vi "Monitor.vi"() -> ()   [LabVIEW 2019]
uses:
  <instrlib>/Siemens ELAN/Message Header.ctl
  <instrlib>/Siemens ELAN/Channel Status.ctl
  <instrlib>/Siemens ELAN/Unit Dimensions.ctl
  <instrlib>/Siemens ELAN/Measured variables.ctl
  <instrlib>/Siemens ELAN/Siemens ELAN.lvlib
panel:
  out "Measured variable":T1
  in  "Source Address":u8=208 format="%.0x"
  in  "Target Address":u8=16 format="%.0x"
  in  "New Name":string
  in  "VISA resource name":refnum<visa-resource-name>="OXYMAT"
  in  "Set Clock":bool
  in  "VISA Timeout Value":u32=200
  out "Channel Name":string
  out "Measurement":cluster{"Measured value":dbl, "Dimension":T2}={"Measured value"=nan, "Dimension"=enum."Unknown (0)"} {"Measured value" format="%#_6f"}
  in  "Broadcast ON?":bool
  out "Maintenance Requests":T3(array[ring])
  in  "Reset":bool
  in  "Remote ON?":bool
  in  "Maintenance ON?":bool
  out "Faults/Errors":T4(array[ring])
  out "time stamp":timestamp format="%<%Y-%m-%dT%H:%M:%S>T"
  out "Channel":T5
  out "Channel Type":T6(ring)
  out "x-y":u32
  in  "milliseconds to wait":u32
  in  "stop":bool
  out "Success":bool
  out "Message Header":T7 {"Source Address" format="%.0x"; "Target Address" format="%.0x"}
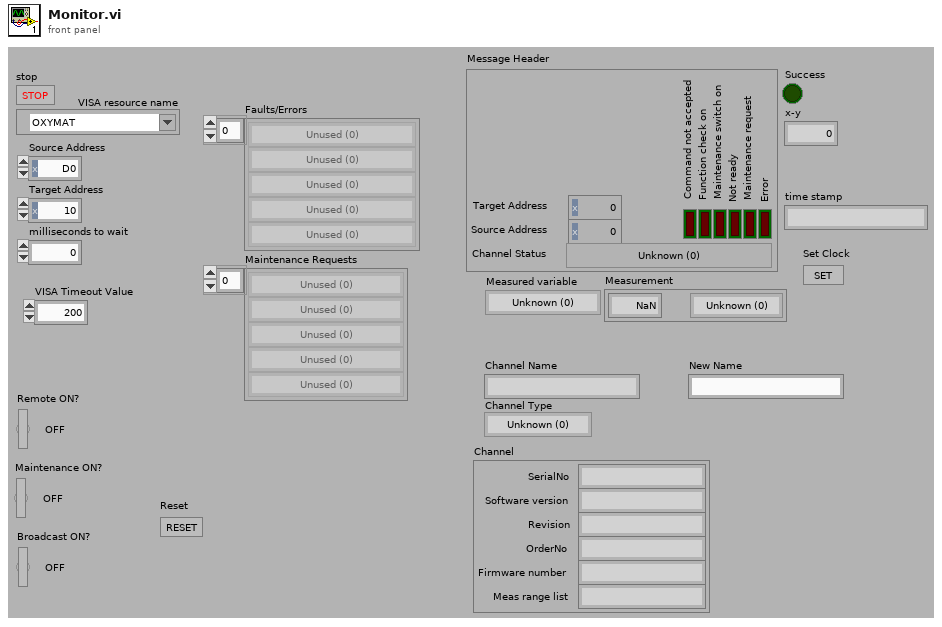
[diagram p1: front panel]
types:
  T1 = typedef "Siemens ELAN.lvlib/Measured variables.ctl" = enum8{"Unknown (0)", "No component", "CO", "CO2", "CH4", "C6H14", "SO2", "NO", "NO2", "CHClF2 (R22)", "C3H8", "C4H10", "O2", "C5H12", "HC", "Pressure", "pH", "Temperature", "C2H4", "C2H2", "C3H6", "C4H6", "C4H8", "C2H6", "NH3", "N2O", "C6H6", "SF6", "CH3OH", "C2H5OH", "CH2Cl2", "C2H4Cl2", "CH3Cl", "C2H4O", "H2O (vapor)", "G/l", "Unknown (36)", "Unknown (37)", "Unknown (38)", "Unknown (39)", "Unknown (40)", "Unknown (41)", "Unknown (42)", "Unknown (43)", "Unknown (44)", "Unknown (45)", "Unknown (46)", "Unknown (47)", "Unknown (48)", "Unknown (49)", "Unknown (50)", "Unknown (51)", "Unknown (52)", "Unknown (53)", "Unknown (54)", "Unknown (55)", "Unknown (56)", "Unknown (57)", "Unknown (58)", "Unknown (59)", "Unknown (60)", "Unknown (61)", "Unknown (62)", "Unknown (63)", "Unknown (64)", "Unknown (65)", "Unknown (66)", "Unknown (67)", "Unknown (68)", "Unknown (69)", "Unknown (70)", "Unknown (71)", "Unknown (72)", "Unknown (73)", "Unknown (74)", "Unknown (75)", "Unknown (76)", "Unknown (77)", "Unknown (78)", "Unknown (79)", "Unknown (80)", "Unknown (81)", "Unknown (82)", "Unknown (83)", "Unknown (84)", "Unknown (85)", "Unknown (86)", "Unknown (87)", "Unknown (88)", "Unknown (89)", "Unknown (90)", "Unknown (91)", "Unknown (92)", "Unknown (93)", "Unknown (94)", "Unknown (95)", "Unknown ((96)", "Unknown (97)", "Unknown (98)", "Unknown (99)", "Ambient Pressure", "Unknown (>100)"}
  T2 = typedef "Siemens ELAN.lvlib/Unit Dimensions.ctl" = enum8{"Unknown (0)", "Pure number", "ppm", "ppb", "vpm", "vpm C1", "vpm C3", "vpm C6", "mg C/m^3", "mg/m^3", "%", "% v/v", "% of range", "% saturation", "%/°C", "%/K", "% w/w", "mV/pH", "mV/mbar", "nA/mbar", "S/m", "S/cm", "mS/m", "mS/cm", "uS/m", "uS/cm", "s", "min", "hr", "pA", "mA", "uV", "mV", "V", "mbar", "hPa", "ml/min", "kohm", "MOhm", "S", "°C", "Hz", "pH", "ug/l", "mg/l", "l/min", "uA", "mg/dm^3", "kPa", "kohm*cm", "MOhm*cm", "°", "Unknown (>51)"}
  T3 = enum8{"Unused (0)", "Cal Tolerance Violated", "Signal Too High With Zero Adj", "Signal Too Low With Span", "Set Clock", "Microflow Sensor Drift", "Display Temperature", "Analyzer Temperature", "Measuring Head Temperature", "External Request"}[]
  T4 = enum8{"Unused (0)", "Param Memory", "Chopper/Magnetic Field", "Microflow Sensor", "External Fault", "AnalyzerTemperature", "Field Device Heater", "Measuring Head Temperature", "Pressure Sensor", "Signal Too Large", "Unused (S10)", "Reference Gas Supply", "Main Power", "Unused (S13)", "Measured Value > Full Scale", "Calibration Aborted", "Low Sample Flow "}[]
  T5 = cluster{"SerialNo":string, "Software version":string, "Revision":string, "OrderNo":string, "Firmware number":string, "Meas range list":string}
  T6 = enum8{"Unknown (0)", "ULTRAMAT 6", "OXYMAT 6", "FIDAMAT 6", "ULTRAMAT 23", "SIPAN 34", "Unknown (6)", "CALOMAT 6", "Unknown (>7)"}
  T7 = typedef "Siemens ELAN.lvlib/Message Header.ctl" = cluster{"Target Address":u8, "Source Address":u8, "Error":bool, "Maintenance request":bool, "Not ready":bool, "Maintenance switch on":bool, "Function check on":bool, "Command not accepted":bool, "Channel Status":T8}
  T8 = typedef "Siemens ELAN.lvlib/Channel Status.ctl" = enum8{"Unknown (0)", "Warm-up", "Pause", "Standby", "Measure", "Zero calibration", "Adjust component slope", "Unknown (7)", "Adjust curve dip", "Adjust linearization sensitivity", "Adjust temperature compensation", "Adjust pressure compensation", "Adjust linearization zero", "Adjust flow sensor", "Autocal", "Adjust phase", "Zero calibration of O2 sensor", "Synchronous zero calibration", "Purging for synchronous zero calibration", "Adjust analog output", "Adjust analog input", "Cleaning", "Unknown (>21)"}
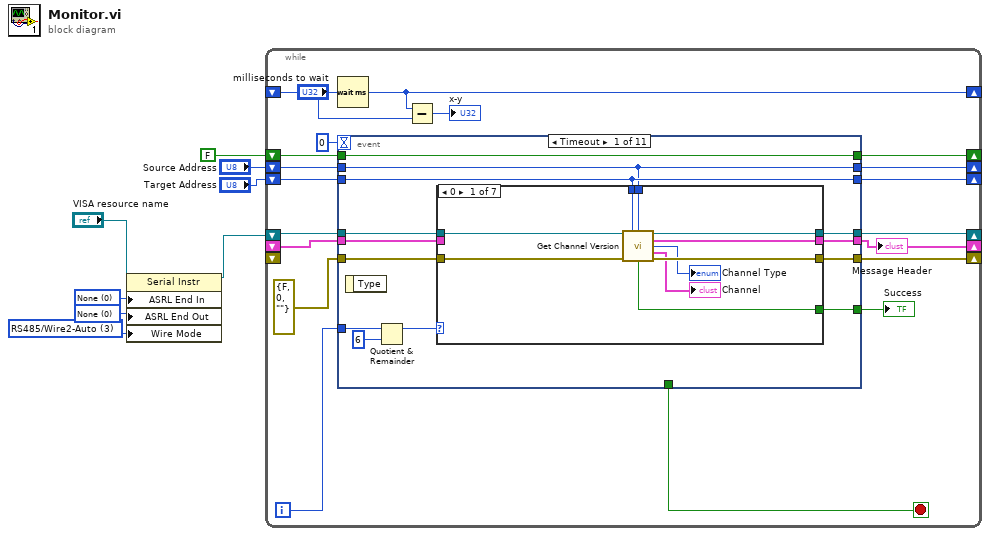
[diagram p0: block diagram]
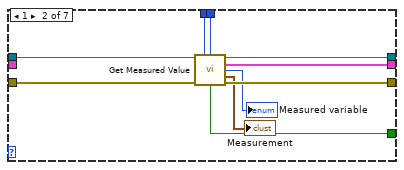
[diagram p2: hidden frame]
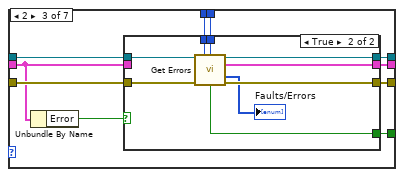
[diagram p3: hidden frame]
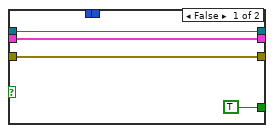
[diagram p4: hidden frame]
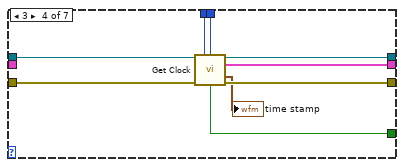
[diagram p5: hidden frame]
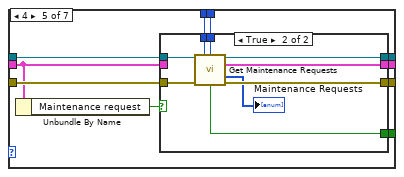
[diagram p6: hidden frame]
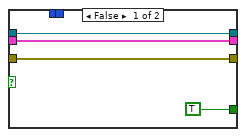
[diagram p7: hidden frame]
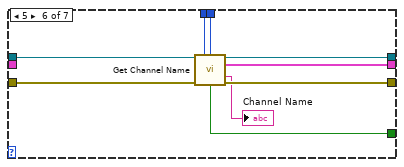
[diagram p8: hidden frame]
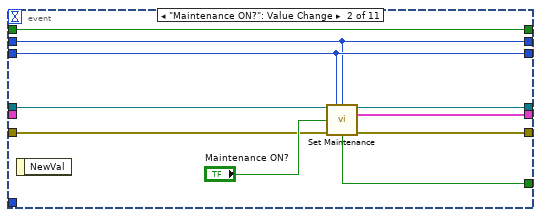
[diagram p10: hidden frame]
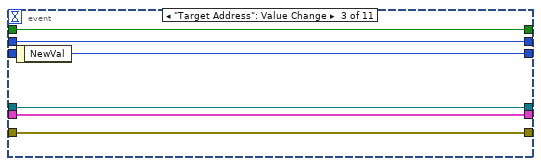
[diagram p11: hidden frame]
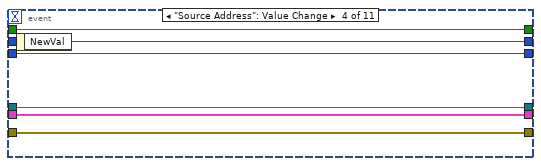
[diagram p12: hidden frame]
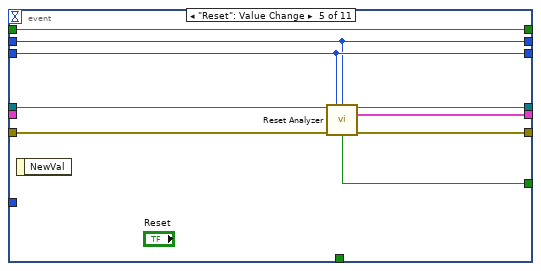
[diagram p13: hidden frame]
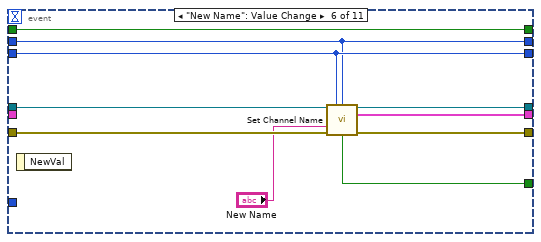
[diagram p14: hidden frame]
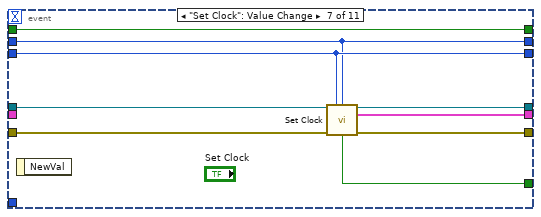
[diagram p15: hidden frame]
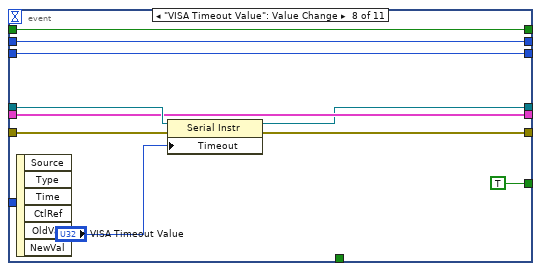
[diagram p16: hidden frame]
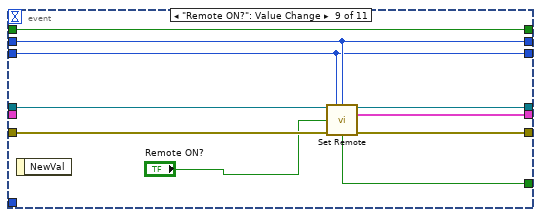
[diagram p17: hidden frame]
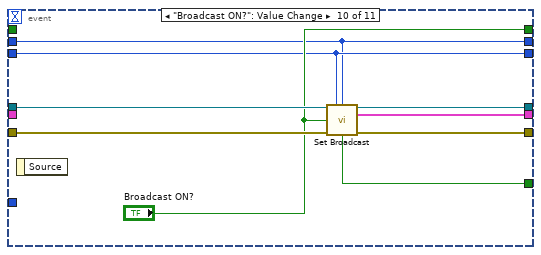
[diagram p18: hidden frame]
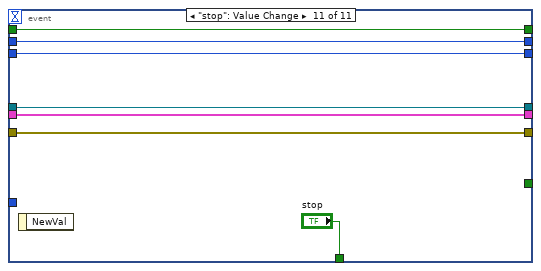
[diagram p19: hidden frame]
diagram:
  w3 = u16 0 items=["None", "Last Bit", "TermChar"] ("Serial Settings:End Mode for Reads")
  w4 = u16 0 items=["None", "Last Bit", "TermChar", "Break"] ("Serial Settings:End Mode for Writes")
  w5 = i16 3 items=["Unknown"=-1, "RS485/Wire4"=0, "RS485/Wire2-EchoDTR"=1, "RS485/Wire2-CtrlDTR"=2, "RS485/Wire2-Auto"=3, "RS232/DTE"=128, "RS232/DCE"=129, "RS232/AUTO"=130] ("Serial Settings:Wire Mode")
  n1 = property class="Serial Instr"(reference="VISA resource name", "ASRL End In"=w3, "ASRL End Out"=w4, "Wire Mode"=w5) -> (reference out=w6:refnum<visa-resource-name>)  [unwired: 1 in, 1 out]
  n2 = while {
    shift-right: [w22] -> _
    shift-left: w6 -> [w24]
    shift-right: [w23] -> _
    shift-left: _ -> [_]
    shift-right: [w28] -> _
    shift-left: _ -> [w27]
    shift-right: [w16] -> _
    shift-left: _ -> [w15]
    shift-right: [w13] -> _
    shift-left: FALSE -> [w14]
    shift-right: [w10] -> _
    shift-left: "Source Address" -> [w12]
    shift-right: [w9] -> _
    shift-left: "Target Address" -> [w11]
    i -> [w17]
    stop <- w20 stop-if-true
    n3 = Wait (ms)(milliseconds to wait="milliseconds to wait") -> (millisecond timer value=w28:u32)
    n4 = event shown="[0] Timeout" {
      selector: _ -> [_ _ _ _ _ _ _ _ _ _ _]
      dyn-events: _ -> [_ _ _ _ _ _ _ _ _ _ _]
      timeout: 0 -> [_ _ _ _ _ _ _ _ _ _ _]
      tunnel: w24 -> [w38 w137 w143 w149 w159 w169 w178 w187 w198 w207 w213]
      tunnel: errorcluster {"status"=FALSE, "code"=0, "source"=""} ("error out") -> [w36 w136 w142 w148 w158 w168 w177 w184 w197 w206 w212]
      tunnel: [w35 w134 w142 w148 w155 w165 w174 w182 w194 w204 w212] -> w23
      tunnel: [w37 w135 w143 w149 w157 w167 w176 w183 w196 w205 w213] -> w22
      tunnel: [_ _ _ _ _ _ _ _ _ _ "stop"] -> w20
      tunnel: w17 -> [w41 _ _ _ _ _ _ _ _ _ _]
      tunnel: [w34 w133 w141 w147 w156 w166 w175 w186 w195 w203 w211] -> w16
      tunnel: [w33 w132 _ _ w154 w164 w173 TRUE ("Success") w193 w202 _] -> w19
      tunnel: w15 -> [w32 _ w141 w147 _ _ _ w186 _ _ w211]
      tunnel: [w31 w131 w144 w150 w153 w163 w172 w188 w191 "Broadcast ON?" w210] -> w13
      tunnel: w14 -> [w31 w131 w144 w150 w153 w163 w172 w188 w191 _ w210]
      tunnel: w12 -> [w29 w129 w140 _ w151 w160 w170 w179 w190 w199 w208]
      tunnel: w11 -> [w30 w130 _ w145 w152 w161 w171 w180 w189 w200 w209]
      tunnel: [w29 w129 w140 w146 w151 w160 w170 w179 w190 w199 w208] -> w10
      tunnel: [w30 w130 w139 w145 w152 w161 w171 w180 w189 w200 w209] -> w9
      event Timeout {
        n5 = event-data() -> ()  [unwired: 1 in, 1 out]
        n6 = Quotient & Remainder(x=w41, y=6) -> (x-y*floor(x/y)=w39:i32)  [unwired: 1 out]
        n7 = case shown="0" w39 {
          tunnel: w38 -> [w49 w61 w69 w93 w103 w125 w128]
          tunnel: [w48 w60 w68 w90 w101 w123 w128] -> w37
          tunnel: w36 -> [w47 w59 w71 w92 w102 w124 w127]
          tunnel: [w51 w58 w70 w91 w99 w121 w127] -> w35
          tunnel: [w46 w57 w67 w88 w100 w122 w126] -> w34
          tunnel: [w45 w56 w66 w87 w98 w120 _] -> w33
          tunnel: w32 -> [_ _ w64 _ w96 _ w126]
          tunnel: w30 -> [w43 w54 w63 w86 w95 w118 _]
          tunnel: w29 -> [w42 w53 w62 w85 w94 w117 _]
          frame 0 {
            n8 = call <instrlib>:"Get Channel Version.vi"("VISA Session In"=w49, "Target Address"=w43, "Source Address"=w42, "error in (no error)"=w47) -> ("VISA Session Out"=w48:refnum<visa-resource-name>, "Message Header"=w46:T7, "Channel Type"=→"Channel Type":T6, "Channel"=→"Channel":T5, "Success"=w45:bool, "error out"=w51:errorcluster)  [unwired: 6 in]
          }
          frame 1 {
            n9 = call <instrlib>:"Get Measured Value.vi"("VISA Session In"=w61, "Target Address"=w54, "Source Address"=w53, "error in (no error)"=w59) -> ("VISA Session Out"=w60:refnum<visa-resource-name>, "Message Header"=w57:T7, "Measured variable"=→"Measured variable":T1, "Measurement"=→"Measurement":cluster{"Measured value":dbl, "Dimension":T2}, "Success"=w56:bool, "error out"=w58:errorcluster)  [unwired: 6 in]
          }
          frame 2 {
            n10 = Unbundle By Name(w64) -> ("Error"=w65:bool)
            n11 = case shown="True" w65 {
              tunnel: w71 -> [w75 w84]
              tunnel: [w75 w83] -> w70
              tunnel: w69 -> [w73 w82]
              tunnel: [w73 w81] -> w68
              tunnel: [w74 w80] -> w67
              tunnel: [TRUE ("Success") w78] -> w66
              tunnel: w64 -> [w74 _]
              tunnel: w63 -> [_ w77]
              tunnel: w62 -> [_ w76]
              frame False {
              }
              frame True {
                n12 = call <instrlib>:"Get Errors.vi"("VISA Session In"=w82, "Target Address"=w77, "Source Address"=w76, "error in (no error)"=w84) -> ("VISA Session Out"=w81:refnum<visa-resource-name>, "Message Header"=w80:T7, "Faults/Errors"=→"Faults/Errors":T4, "Success"=w78:bool, "error out"=w83:errorcluster)  [unwired: 7 in]
              }
            }
          }
          frame 3 {
            n13 = call <instrlib>:"Get Clock.vi"("VISA Session In"=w93, "Target Address"=w86, "Source Address"=w85, "error in (no error)"=w92) -> ("VISA Session Out"=w90:refnum<visa-resource-name>, "Message Header"=w88:T7, "time stamp"=→"time stamp":timestamp, "Success"=w87:bool, "error out"=w91:errorcluster)  [unwired: 7 in]
          }
          frame 4 {
            n14 = Unbundle By Name(w96) -> ("Maintenance request"=w97:bool)
            n15 = case shown="True" w97 {
              tunnel: w103 -> [w106 w116]
              tunnel: w102 -> [w107 w115]
              tunnel: [w106 w114] -> w101
              tunnel: [w105 w113] -> w100
              tunnel: [w107 w112] -> w99
              tunnel: [TRUE ("Success") w111] -> w98
              tunnel: w96 -> [w105 _]
              tunnel: w95 -> [_ w109]
              tunnel: w94 -> [_ w108]
              frame False {
              }
              frame True {
                n16 = call <instrlib>:"Get Maintenance Requests.vi"("VISA Session In"=w116, "Target Address"=w109, "Source Address"=w108, "error in (no error)"=w115) -> ("VISA Session Out"=w114:refnum<visa-resource-name>, "Message Header"=w113:T7, "Maintenance Requests"=→"Maintenance Requests":T3, "Success"=w111:bool, "error out"=w112:errorcluster)  [unwired: 7 in]
              }
            }
          }
          frame 5 {
            n17 = call <instrlib>:"Get Channel Name.vi"("VISA Session In"=w125, "Target Address"=w118, "Source Address"=w117, "error in (no error)"=w124) -> ("VISA Session Out"=w123:refnum<visa-resource-name>, "Message Header"=w122:T7, "Channel Name"=→"Channel Name":string, "Success"=w120:bool, "error out"=w121:errorcluster)  [unwired: 7 in]
          }
          frame Default {
          }
        }
      }
      event "Maintenance ON?": Value Change {
        n18 = event-data() -> ()  [unwired: 1 in, 1 out]
        n19 = call <instrlib>:"Set Maintenance.vi"("VISA Session In"=w137, "Target Address"=w130, "Source Address"=w129, "Maintenance ON?"="Maintenance ON?", "error in (no error)"=w136) -> ("VISA Session Out"=w135:refnum<visa-resource-name>, "Message Header"=w133:T7, "Success"=w132:bool, "error out"=w134:errorcluster)  [unwired: 7 in]
      }
      event "Target Address": Value Change {
        n20 = event-data() -> ("NewVal"=w139:u8)  [unwired: 1 in]
      }
      event "Source Address": Value Change {
        n21 = event-data() -> ("NewVal"=w146:u8)  [unwired: 1 in]
      }
      event "Reset": Value Change {
        n22 = event-data() -> ()  [unwired: 1 in, 1 out]
        n23 = call <instrlib>:"Reset Analyzer.vi"("VISA Session In"=w159, "Target Address"=w152, "Source Address"=w151, "error in (no error)"=w158) -> ("VISA Session Out"=w157:refnum<visa-resource-name>, "Message Header"=w156:T7, "Success"=w154:bool, "error out"=w155:errorcluster)  [unwired: 8 in]
      }
      event "New Name": Value Change {
        n24 = event-data() -> ()  [unwired: 1 in, 1 out]
        n25 = call <instrlib>:"Set Channel Name.vi"("VISA Session In"=w169, "Target Address"=w161, "Source Address"=w160, "Channel Name"="New Name", "error in (no error)"=w168) -> ("VISA Session Out"=w167:refnum<visa-resource-name>, "Message Header"=w166:T7, "Success"=w164:bool, "error out"=w165:errorcluster)  [unwired: 7 in]
      }
      event "Set Clock": Value Change {
        n26 = event-data() -> ()  [unwired: 1 in, 1 out]
        n27 = call <instrlib>:"Set Clock.vi"("VISA Session In"=w178, "Target Address"=w171, "Source Address"=w170, "error in (no error)"=w177) -> ("VISA Session Out"=w176:refnum<visa-resource-name>, "Message Header"=w175:T7, "Success"=w173:bool, "error out"=w174:errorcluster)  [unwired: 8 in]
      }
      event "VISA Timeout Value": Value Change {
        n28 = event-data() -> ()  [unwired: 1 in, 6 out]
        n29 = property class="Serial Instr"(reference=w187, error in=w184, "Timeout"="VISA Timeout Value") -> (reference out=w183:refnum<visa-resource-name>, error out=w182:errorcluster)
      }
      event "Remote ON?": Value Change {
        n30 = event-data() -> ()  [unwired: 1 in, 1 out]
        n31 = call <instrlib>:"Set Remote.vi"("VISA Session In"=w198, "Target Address"=w189, "Source Address"=w190, "Remote ON?"="Remote ON?", "error in (no error)"=w197) -> ("VISA Session Out"=w196:refnum<visa-resource-name>, "Message Header"=w195:T7, "Success"=w193:bool, "error out"=w194:errorcluster)  [unwired: 7 in]
      }
      event "Broadcast ON?": Value Change {
        n32 = event-data() -> ()  [unwired: 1 in, 1 out]
        n33 = call <instrlib>:"Set Broadcast.vi"("VISA Session In"=w207, "Target Address"=w200, "Source Address"=w199, "Broadcast ON?"="Broadcast ON?", "error in (no error)"=w206) -> ("VISA Session Out"=w205:refnum<visa-resource-name>, "Message Header"=w203:T7, "Success"=w202:bool, "error out"=w204:errorcluster)  [unwired: 7 in]
      }
      event "stop": Value Change {
        n34 = event-data() -> ()  [unwired: 1 in, 1 out]
      }
    }
    "Message Header" <- w16
    "Success" <- w19
    n35 = Subtract(x=w28, y=w27) -> (x-y=→"x-y":u32)
  }
